vi "SV Peak Hold Spectra (Real).vi"(0 "real spectra":cluster{"f0":dbl, "df":dbl, "magnitude":dbl[]}[](array[cluster]) {"magnitude" format="%.2p"; "df" format="%.2p"; "f0" format="%.2p"}, 4 "spectrum info":T1={"channel name"="", "description"="", "x-axis units"=0, "spectral info"={"spectrum type"=enum."Power [Magnitude^2]", "linear/dB"=enum."linear", "window"=0, "window size"=0, "FFT size"=0}, "engineering units"=1, "custom label"="", "dB reference [EU]"=0.0, "peak units"=enum."rms", "weighting filter"=0, "spectral density?"=FALSE, "unit label"="", "spectrum skewed?"=FALSE, "complimentary spectrum units"=enum."none"} {"x-axis units" items=["Time (s)"=0, "Frequency-CB (Hz)"=1, "Frequency-CPB (Hz)"=1248, "Frequency-Arbitrary (Hz)"=2357, "Quefrency (s)"=2, "Revolutions (rev)"=3, "Order"=4, "Speed (RPM)"=11, "Speed (rad/s)"=21, "Index"=65535]; "weighting filter" items=["Linear", "A-weighting", "B-weighting", "C-weighting", "ITU-R 468-4", "Dolby", "CCITT", "C-message", "Wb", "Wc", "Wd", "We", "Wf", "Wh", "Wj", "Wk", "Wm", "AES17 20 kHz lowpass", "AES17 40 kHz lowpass", "AES17 20 kHz highpass", "AES17 40 kHz highpass"]; "dB reference [EU]" format="%.2f"; "engineering units" items=["custom..."=0, "V"=1, "A"=21, "C"=30, "pC"=31, "s"=32, "-"=29, "Pa"=2, "N"=20, "g"=3, "m/s^2"=4, "m/s"=5, "m"=6, "mm/s"=12, "mm"=13, "micron/s"=14, "micron"=15, "in/s^2"=7, "in/s"=8, "in"=9, "mil/s"=10, "mil"=11, "rad/s^2"=16, "rad/s"=17, "rad"=18, "deg/s^2"=26, "deg/s"=27, "deg"=28, "RPM"=22, "cycle/s^2"=23, "Hz"=24, "cycle"=25, "strain"=19]; "spectral info"."window" items=["None "=0, "Hanning"=1, "Hamming"=2, "Blackman-Harris"=3, "Exact Blackman"=4, "Blackman"=5, "Flat Top"=6, "4 Term B-Harris "=7, "7 Term B-Harris"=8, "Low Sidelobe"=9, "Force - Exponential"=10, "Gaussian"=62]}, 5 "error in (no error)":errorcluster) -> (13 "averages completed":dbl, 14 "peak hold spectrum":cluster{"f0":dbl, "df":dbl, "magnitude":dbl[]} {"magnitude" format="%.2p"; "df" format="%.2p"; "f0" format="%.2p"}, 15 "unit label":string, 18 "spectrum info":T1={"channel name"="", "description"="", "x-axis units"=0, "spectral info"={"spectrum type"=enum."Power [Magnitude^2]", "linear/dB"=enum."linear", "window"=0, "window size"=0, "FFT size"=0}, "engineering units"=1, "custom label"="", "dB reference [EU]"=0.0, "peak units"=enum."rms", "weighting filter"=0, "spectral density?"=FALSE, "unit label"="", "spectrum skewed?"=FALSE, "complimentary spectrum units"=enum."none"} {"x-axis units" items=["Time (s)"=0, "Frequency-CB (Hz)"=1, "Frequency-CPB (Hz)"=1248, "Frequency-Arbitrary (Hz)"=2357, "Quefrency (s)"=2, "Revolutions (rev)"=3, "Order"=4, "Speed (RPM)"=11, "Speed (rad/s)"=21, "Index"=65535]; "weighting filter" items=["Linear", "A-weighting", "B-weighting", "C-weighting", "ITU-R 468-4", "Dolby", "CCITT", "C-message", "Wb", "Wc", "Wd", "We", "Wf", "Wh", "Wj", "Wk", "Wm", "AES17 20 kHz lowpass", "AES17 40 kHz lowpass", "AES17 20 kHz highpass", "AES17 40 kHz highpass"]; "dB reference [EU]" format="%.2f"; "engineering units" items=["custom..."=0, "V"=1, "A"=21, "C"=30, "pC"=31, "s"=32, "-"=29, "Pa"=2, "N"=20, "g"=3, "m/s^2"=4, "m/s"=5, "m"=6, "mm/s"=12, "mm"=13, "micron/s"=14, "micron"=15, "in/s^2"=7, "in/s"=8, "in"=9, "mil/s"=10, "mil"=11, "rad/s^2"=16, "rad/s"=17, "rad"=18, "deg/s^2"=26, "deg/s"=27, "deg"=28, "RPM"=22, "cycle/s^2"=23, "Hz"=24, "cycle"=25, "strain"=19]; "spectral info"."window" items=["None "=0, "Hanning"=1, "Hamming"=2, "Blackman-Harris"=3, "Exact Blackman"=4, "Blackman"=5, "Flat Top"=6, "4 Term B-Harris "=7, "7 Term B-Harris"=8, "Low Sidelobe"=9, "Force - Exponential"=10, "Gaussian"=62]}, 19 "error out":errorcluster)   [LabVIEW 2017]
doc: "Computes the linear RMS-averaged power spectrum of <B>scaled signal [EU]</B> in a linear scale. Use the power spectrum to quantify signal components as a function of frequency. Use this VI on embedded targets that have limited computational resources. Wire data to the <B>scaled signal [EU]</B> input to determine the polymorphic instance to use or manually select the instance."
uses:
  <vilib>/addons/_NISVFA/_Shared subVIs/Controls/svc_Spectrum Info.ctl
  <vilib>/addons/_NISVFA/_Shared subVIs/Controls/svc_X-Axis Units.ctl
  <vilib>/addons/_NISVFA/_Shared subVIs/Controls/svc_Spectrum Type.ctl
  <vilib>/addons/_NISVFA/_Shared subVIs/Controls/svc_Engineering Units Text Ring.ctl
  <vilib>/addons/_NISVFA/_Shared subVIs/Controls/svc_Weighting Filter Text Ring.ctl
  <vilib>/addons/_NISVFA/_Shared subVIs/Controls/svc_Complimentary Spectrum Units.ctl
  <vilib>/addons/_NISVFA/_Shared subVIs/Common/svc_Get Weighting Enum and Labels.vi
  <vilib>/addons/_NISVFA/_Shared subVIs/Common/svc_Unit Label Lexical Class.vi
  <vilib>/addons/_NISVFA/_Shared subVIs/Common/svc_Engineering Units to Unit Label.vi
  <vilib>/addons/_NISVFA/_Shared subVIs/Common/svc_Format Value (DBL).vi
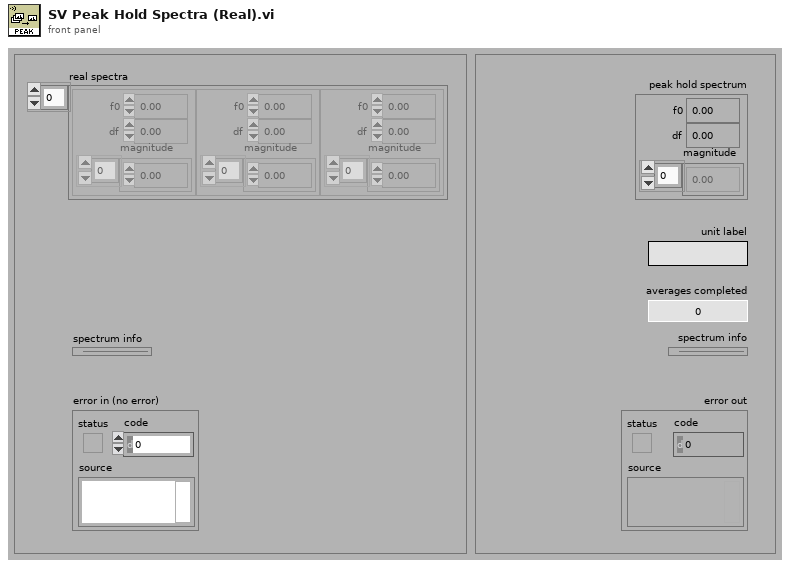
[diagram p1: front panel]
types:
  T1 = typedef "svc_Spectrum Info.ctl" = cluster{"channel name":string, "description":string, "x-axis units":T2, "spectral info":cluster{"spectrum type":T3, "linear/dB":enum16{"linear", "dB"}, "window":u16, "window size":i32, "FFT size":i32}, "engineering units":T4, "custom label":string, "dB reference [EU]":dbl, "peak units":enum16{"rms", "peak", "peak-peak"}, "weighting filter":T5, "spectral density?":bool, "unit label":string, "spectrum skewed?":bool, "complimentary spectrum units":T6}
  T2 = typedef "svc_X-Axis Units.ctl" = u16
  T3 = typedef "svc_Spectrum Type.ctl" = enum16{"FFT Spectrum [complex]", "Amplitude [Magnitude]", "Power [Magnitude^2]", "Cross Spectrum [complex]", "Frequency Response [Complex]"}
  T4 = typedef "svc_Engineering Units Text Ring.ctl" = u16
  T5 = typedef "svc_Weighting Filter Text Ring.ctl" = u16
  T6 = typedef "svc_Complimentary Spectrum Units.ctl" = enum16{"none", "radians", "degrees", "cycles", "imaginary"}
  T7 = enum16{"Restart processing", "Continue processing", "Skip processing"}
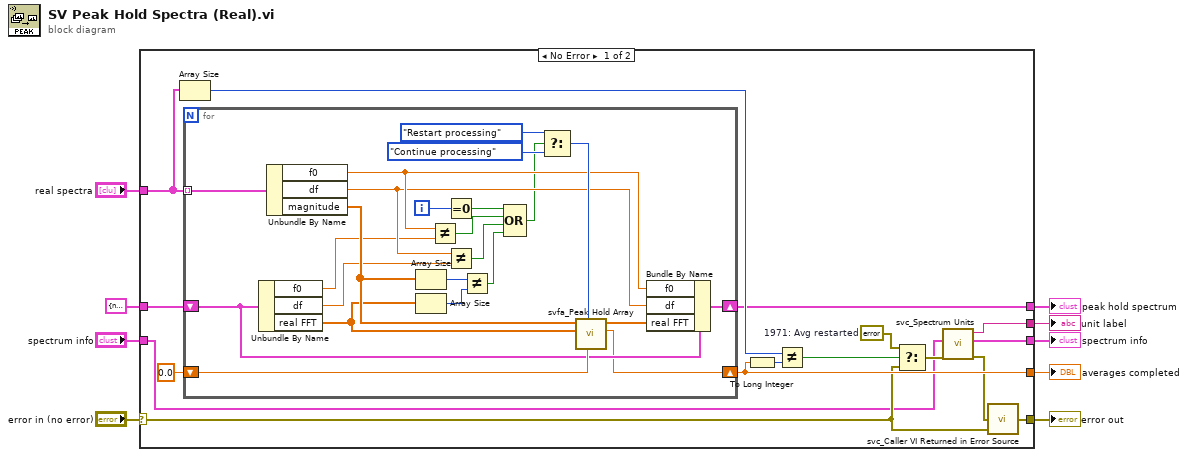
[diagram p0: block diagram]
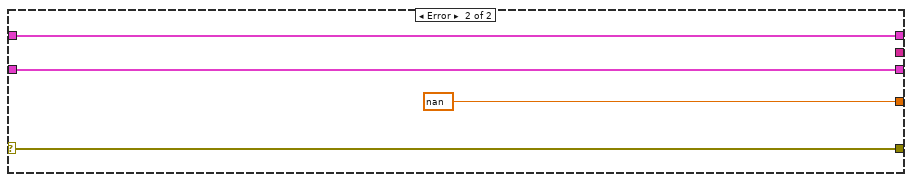
[diagram p2: hidden frame]
diagram:
  n1 = case shown="No Error" "error in (no error)" {
    selector: "error in (no error)" -> [w13 w51]
    tunnel: [w17 w49] -> w9
    tunnel: "real spectra" -> [w18 _]
    tunnel: [w24 nan ("Numeric")] -> w7
    tunnel: "spectrum info" -> [w10 w50]
    tunnel: [w19 w51] -> w4
    tunnel: [w16 w50] -> w3
    tunnel: [w14 _] -> w2
    tunnel: cluster{"f0":dbl, "df":dbl, "real FFT":dbl[]} {"f0"=nan, "df"=nan, "real FFT"=[]} ("previous avg real spectrum") -> [w11 w49]
    frame No Error {
      w21 = errorcluster {"status"=FALSE, "code"=1971, "source"="<append>\n\nPeak Hold restarted due to change in f0, df, or spectrum size within real spectra input."}  # 1971: Avg restarted
      n2 = Array Size(array=w18) -> (size(s)=w23:i32)
      n3 = for {
        tunnel: w18 -> [w26] mode=indexing
        shift-right: [w29] -> w24
        shift-left: 0.0 ("Numeric") -> [w38]
        shift-right: [w31] -> w17
        shift-left: w11 -> [w35]
        i -> [w36]
        n4 = Unbundle By Name(w35) -> ("f0"=w28:dbl, "df"=w27:dbl, "real FFT"=w39:dbl[])
        n5 = Unbundle By Name(w26) -> ("f0"=w33:dbl, "df"=w32:dbl, "magnitude"=w48:dbl[])
        n6 = Array Size(array=w48) -> (size(s)=w47:i32)
        n7 = Array Size(array=w39) -> (size(s)=w46:i32)
        n8 = Not Equal?(x=w33, y=w28) -> (x != y?=w45:bool)
        n9 = Equal To 0?(x=w36) -> (x = 0?=w37:bool)
        n10 = Not Equal?(x=w32, y=w27) -> (x != y?=w41:bool)
        n11 = Not Equal?(x=w47, y=w46) -> (x != y?=w44:bool)
        n12 = Compound Arithmetic op=OR(w37, w45, w41, w44) -> (w30:bool)
        n13 = Select(t=T7."Restart processing", s=w30, f=T7."Continue processing" ("processing control")) -> (s? t:f=w40:T7)
        n14 = call <vilib>:"svfa_Peak Hold Array.vi"("averages completed in"=w38, "processing control"=w40, "previous peak array"=w39, "array"=w48) -> ("averages completed out"=w29:dbl, "peak array"=w34:dbl[])  [unwired: 5 in, 1 out]
        n15 = Bundle By Name(cluster=w35, "f0"=w33, "df"=w32, "real FFT"=w34) -> (w31:cluster{"f0":dbl, "df":dbl, "real FFT":dbl[]})
      }
      n16 = To Long Integer(number=w24) -> (32bit integer=w22:i32)
      n17 = Not Equal?(x=w23, y=w22) -> (x != y?=w20:bool)
      n18 = Select(t=w21, s=w20, f=w13) -> (s? t:f=w12:errorcluster)
      n19 = call <vilib>:"svc_Spectrum Units.vi"("error in (no error)"=w12, "spectrum info in"=w10) -> ("error out"=w15:errorcluster, "spectrum info out"=w16:T1, "unit label"=w14:string)  [unwired: 2 in, 1 out]
      n20 = call <vilib>:"svc_Caller VI Returned in Error Source.vi"("warning input to caller"=w13, "error in (no error)"=w15) -> ("error out"=w19:errorcluster)  [unwired: 3 in]
    }
    frame Error {
    }
  }
  "peak hold spectrum" <- w9
  "averages completed" <- w7
  "error out" <- w4
  "spectrum info" <- w3
  "unit label" <- w2
